vi "receiver.vi"() -> ()   [LabVIEW 2015]
uses:
  <vilib>/addons/Modulation/niDMT.lvlib
  <vilib>/addons/Modulation/Digital/General/MT Generate FSK System Parameters(M).vi
  <instrlib>/niUSRP/niUSRP Fetch Rx Data (CDB Cluster).vi
  <vilib>/addons/Modulation/niAMT.lvlib
  <vilib>/addons/Modulation/Analog/MT Downconvert Passband (Complex).vi
panel:
  in  "passband bandwidth (Hz)":dbl format="%.2p"
  out "XY Graph":T1(graph)
  out "output bit stream":i8[](array[numeric])
  in  "symbol phase continuity":enum16{"continuous", "discontinuous"}(ring)
  in  "symbol rate":dbl
  in  "eye length":i32=3
  in  "active antenna":string
  in  "stop button":bool
  out "RMS FSK Deviation Measurements (Hz)":dbl[](array[numeric])
  out "Eye Diagram":cluster{"t0":dbl, "dt":dbl, "Y":dbl[]}[](graph)
  in  "number of samples":i64=100000
  in  "matched samples per symbol (16)":i32=16
  in  "modulation type":T2(ring)
  in  "pulse shaping filter (none)":T3(ring)
  out "coerced carrier frequency":dbl=100000.0 format="%#_6p"
  out "coerced gain":dbl format="%#_6f"
  out "coerced IQ rate":dbl=100000.0 format="%#_6p"
  in  "gain":dbl format="%#_6f"
  in  "carrier frequency":dbl=100000.0 format="%#_6p"
  in  "IQ rate":dbl=100000.0 format="%#_6p"
  in  "FSK deviation (Hz)":dbl=150000.0 format="%.2p"
  in  "M-FSK (2)":i32=2
  in  "samples per symbol (16)":i32=16
  in  "device names":refnum<k15>
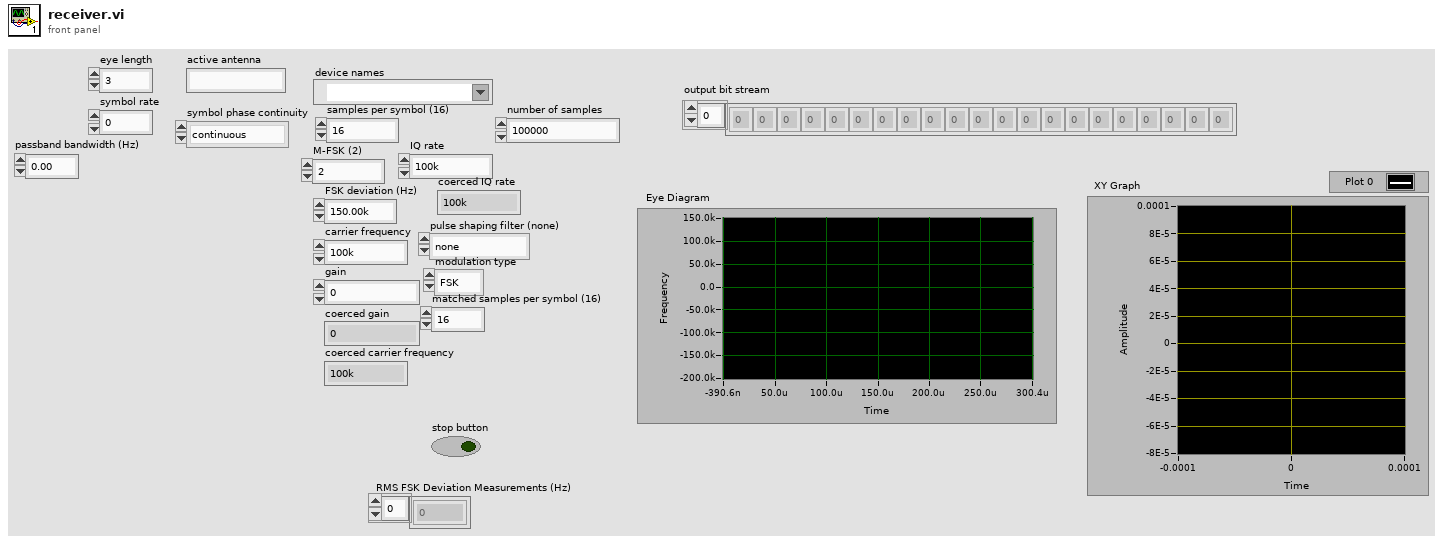
[diagram p1: front panel]
types:
  T1 = cluster{"constellation":dbl[], "oversampled data":dbl[]}[]
  T2 = enum16{"FSK", "PSK", "QAM", "MSK", "PAM", "ASK", "CPM"}
  T3 = enum16{"none", "Raised Cosine", "Root Raised Cos", "Gaussian"}
  T4 = cluster{"samples per symbol (16)":i32, "symbol map":dbl[], "symbol phase continuity":enum16{"continuous", "discontinuous"}}
  T5 = typedef "niAMT.lvlib/Complex Data Waveform.ctl" = cluster{"t0":dbl, "dt":dbl, "Y":cdb[]}
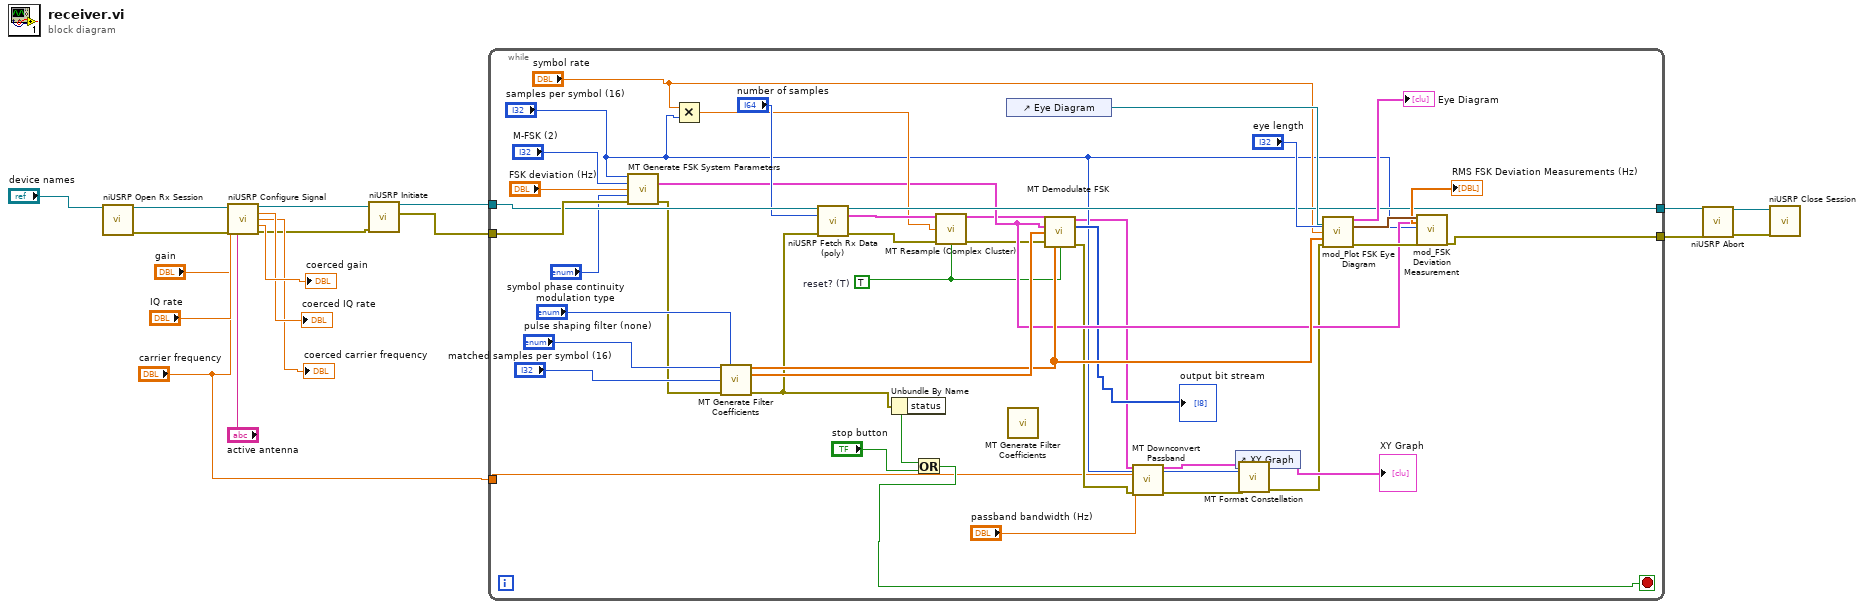
[diagram p0: block diagram]
diagram:
  n1 = call <instrlib>:"niUSRP Open Rx Session.vi"("device names"="device names") -> ("session handle out"=w17:refnum<k15>, "error out"=w16:errorcluster)  [unwired: 13 in]
  n2 = call <instrlib>:"niUSRP Configure Signal.vi"("session handle"=w17, "IQ rate"="IQ rate", "carrier frequency"="carrier frequency", "gain"="gain", "error in (no error)"=w16, "active antenna"="active antenna") -> ("session handle out"=w10:refnum<k15>, "coerced IQ rate"=→"coerced IQ rate":dbl, "coerced carrier frequency"=→"coerced carrier frequency":dbl, "coerced gain"=→"coerced gain":dbl, "error out"=w9:errorcluster)  [unwired: 5 in]
  n3 = call <instrlib>:"niUSRP Initiate.vi"("session handle"=w10, "error in (no error)"=w9) -> ("session handle out"=w7:refnum<k15>, "error out"=w8:errorcluster)  [unwired: 12 in]
  n4 = while {
    tunnel: w8 -> [w59]
    tunnel: w7 -> [w55]
    tunnel: [w37] -> w6
    tunnel: [w43] -> w5
    tunnel: "carrier frequency" -> [w20]
    stop <- w40 stop-if-true
    w25 = TRUE  # reset? (T)
    n5 = call-poly <vilib>:"MT Generate FSK System Parameters.vi"("samples per symbol (16)"="samples per symbol (16)", "M-FSK (2)"="M-FSK (2)", "FSK deviation (Hz)"="FSK deviation (Hz)", "symbol phase continuity"="symbol phase continuity", "error in (no error)"=w59) -> ("FSK system parameters"=w34:T4, "error out"=w53:errorcluster)  [unwired: 9 out]
    n6 = Multiply(x="symbol rate", y="samples per symbol (16)") -> (x*y=w36:dbl)
    n7 = call <vilib>:"MT Generate Filter Coefficients.vi"("pulse shaping filter (none)"="pulse shaping filter (none)", "modulation type"="modulation type", "matched samples per symbol (16)"="matched samples per symbol (16)", "error in (no error)"=w53) -> ("pulse shaping filter coefficients"=w49:dbl[], "matched filter coefficients"=w50:dbl[], "error out"=w39:errorcluster)  [unwired: 3 in, 6 out]
    n8 = call-poly <instrlib>:"niUSRP Fetch Rx Data (poly).vi"("session handle"=w55, "number of samples"="number of samples", "error in (no error)"=w39) -> ("session handle out"=w37:refnum<k15>, "data"=w52:cluster{"t0":dbl, "dt":dbl, "Y":cdb[]}, "error out"=w51:errorcluster)  [unwired: 9 in, 1 out]
    n9 = Unbundle By Name(w39) -> ("status"=w41:bool)
    n10 = Or(x=w41, y="stop button") -> (x .or. y?=w40:bool)
    n11 = call <vilib>:"MT Resample (Complex Cluster).vi"("input complex waveform"=w52, "desired sample rate (Hz)"=w36, "error in (no error)"=w51, "reset? (T)"=w25) -> ("output complex waveform"=w33:T5, "error out"=w30:errorcluster)  [unwired: 2 in, 8 out]
    n12 = control-ref of="Eye Diagram"() -> (w48:refnum<vi>)
    n13 = call <vilib>:"MT Generate Filter Coefficients.vi"() -> ()  [unwired: 13 in, 3 out]
    n14 = call <vilib>:"MT Demodulate FSK.vi"("input complex waveform"=w33, "FSK system parameters"=w34, "matched filter coefficients"=w50, "error in (no error)"=w30, "pulse shaping filter coefficients"=w49, "reset? (T)"=w25) -> ("recovered complex waveform"=w23:T5, "output bit stream"=→"output bit stream":i8[], "error out"=w24:errorcluster)  [unwired: 1 in, 6 out]
    n15 = call-poly <vilib>:"MT Downconvert Passband.vi"("complex waveform"=w23, "carrier frequency (Hz)"=w20, "passband bandwidth (Hz)"="passband bandwidth (Hz)", "error in (no error)"=w24) -> ("downconverted waveform (complex)"=w21:T5, "error out"=w22:errorcluster)  [unwired: 8 in, 2 out]
    n16 = control-ref of="XY Graph"() -> (w26:refnum<vi>)
    n17 = call <vilib>:"MT Format Constellation.vi"("waveform"=w21, "constellation reference"=w26, "samples per symbol"="samples per symbol (16)", "error in (no error)"=w22) -> ("constellation graph"=→"XY Graph":T1, "error out"=w28:errorcluster)  [unwired: 10 in]
    n18 = call <vilib>:"mod_Plot FSK Eye Diagram.vi"("Rx Eye Diagram"=w48, "eye length"="eye length", "Symbol Rate, Hz"="symbol rate", "matched filter coefficients"=w49, "error in (no error)"=w28) -> ("FSK Eye Diagram"=→"Eye Diagram":cluster{"t0":dbl, "dt":dbl, "Y":dbl[]}[], "output FM demodulated waveform"=w47:waveform(dbl), "error out"=w44:errorcluster)  [unwired: 3 in, 5 out]
    n19 = call <vilib>:"mod_FSK Deviation Measurement.vi"("FM demodulated waveform in"=w47, "FSK system parameters"=w34, "samples per symbol (16)"="samples per symbol (16)", "error in (no error)"=w44) -> ("RMS FSK Deviation Measurements (Hz)"=→"RMS FSK Deviation Measurements (Hz)":dbl[], "error out"=w43:errorcluster)  [unwired: 14 out]
  }
  n20 = call <instrlib>:"niUSRP Abort.vi"("session handle"=w6, "error in (no error)"=w5) -> ("session handle out"=w4:refnum<k15>, "error out"=w3:errorcluster)  [unwired: 12 in]
  n21 = call <instrlib>:"niUSRP Close Session.vi"("session handle"=w4, "error in (no error)"=w3) -> ()  [unwired: 13 in, 1 out]
